vi "setParamsAcq.vi"(0 "Acquisition in":refnum<class "Acquisition.lvclass">, 5 "Params":T1={"Mice ID"=[], "ExpType"=[], "Trial Interval"=[], "Pulse Duration"=[158.0, 152.0, 156.0, 167.0, 172.0], "microL_per_pulse"=[6.0, 6.0, 6.0, 6.0, 6.0], "Response Interval"=[1000.0, 1000.0, 1000.0, 1000.0, 1000.0], "Bad Delay"=[], "Response Period"=[], "liquid_type"="water", "Stimuli"=[], "Rewarded Stimuli"=[]}, 11 "error in (no error)":errorcluster) -> (4 "Acquisition out":refnum<class "Acquisition.lvclass">, 15 "error out":errorcluster)   [LabVIEW 2014, in "Acquisition.lvclass"]
uses:
  Acquisition.lvclass
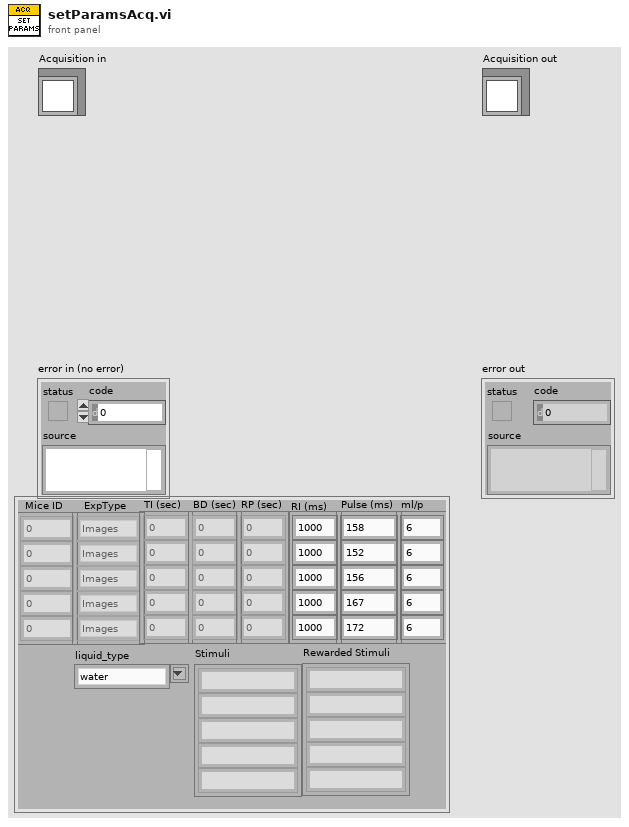
[diagram p1: front panel]
types:
  T1 = cluster{"Mice ID":dbl[], "ExpType":enum16{"Images", "Orientation", "Calibrate", "Freerun", "BW"}[], "Trial Interval":dbl[], "Pulse Duration":dbl[], "microL_per_pulse":dbl[], "Response Interval":dbl[], "Bad Delay":dbl[], "Response Period":dbl[], "liquid_type":string, "Stimuli":string[], "Rewarded Stimuli":string[]}
  T2 = enum16{"Images", "Orientation", "Calibrate", "Freerun", "BW"}[]
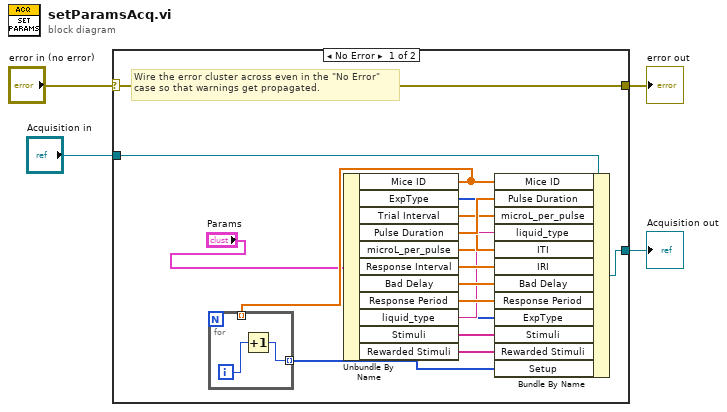
[diagram p0: block diagram]
diagram:
  n1 = case shown="No Error" "error in (no error)" {
    selector: "error in (no error)" -> [w20 w24]
    tunnel: [w20 w24] -> w3
    tunnel: [w18 w23] -> w1
    tunnel: "Acquisition in" -> [w19 w23]
    frame No Error {
      # "Wire the error cluster across even in the \"No Error\"\ncase so that warnings get propagated."
      n2 = Unbundle By Name("Params") -> ("Mice ID"=w8:dbl[], "ExpType"=w5:T2, "Trial Interval"=w16:dbl[], "Pulse Duration"=w17:dbl[], "microL_per_pulse"=w12:dbl[], "Response Interval"=w15:dbl[], "Bad Delay"=w13:dbl[], "Response Period"=w14:dbl[], "liquid_type"=w11:string, "Stimuli"=w10:string[], "Rewarded Stimuli"=w9:string[])
      n3 = for {
        tunnel: w8 -> [_] mode=indexing
        tunnel: [w22] -> w7 mode=indexing
        i -> [w21]
        n4 = Increment(x=w21) -> (x+1=w22:i32)
      }
      n5 = Bundle By Name(cluster=w19, "Mice ID"=w8, "Pulse Duration"=w17, "microL_per_pulse"=w12, "liquid_type"=w11, "ITI"=w16, "IRI"=w15, "Bad Delay"=w13, "Response Period"=w14, "ExpType"=w5, "Stimuli"=w10, "Rewarded Stimuli"=w9, "Setup"=w7) -> (w18:refnum<class "Acquisition.lvclass">)
    }
    frame Error {
    }
  }
  "error out" <- w3
  "Acquisition out" <- w1
